vi "ULTRA Align.vi"(1 "Noodle?":bool) -> (0 "Speed":dbl)   [LabVIEW 2014]
uses:
  TypeDefs/SRE Enum.ctl
panel:
  in  "PD Gains":cluster{"P":dbl, "D":dbl}={"P"=0.02, "D"=0.0}
  in  "Set Noodle":dbl=40.0
  in  "Set Load":dbl=83.0
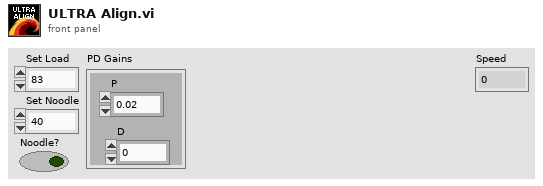
[diagram p1: front panel]
types:
  T1 = typedef "SRE Enum.ctl" = enum16{"Start", "Run", "End"}
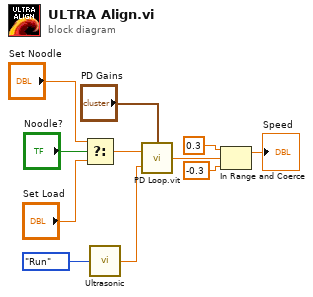
[diagram p0: block diagram]
diagram:
  n1 = Select(t="Set Noodle", s="Noodle?", f="Set Load") -> (s? t:f=w8:dbl)
  n2 = call "Ultrasonic.vi"("Enum"=SRE_Enum."Run") -> ("Distance"=w6:dbl)
  n3 = call "PD Loop.vit"("PD Gains"="PD Gains", "Current"=w6, "Set"=w8) -> ("Out Power"=w2:dbl)
  n4 = In Range and Coerce(upper limit=0.3, x=w2, lower limit=-0.3) -> (coerced(x)=→"Speed":dbl)  [unwired: 1 out]
